vi "Check Mouse In Border Focus.vi"(8 "error in (no error)":errorcluster, 10 "MousePoint":cluster{"x":i16, "y":i16}, 11 "Canvas in":refnum<class "Canvas.lvclass">) -> (0 "error out":errorcluster, 2 "In Border Focus":bool, 3 "Canvas out":refnum<class "Canvas.lvclass">)   [LabVIEW 2015, in "Canvas.lvclass"]
uses:
  Canvas.lvclass
  Canvas.lvclass/Canvas.ctl
  Scalable Border/Scalable Border.lvclass
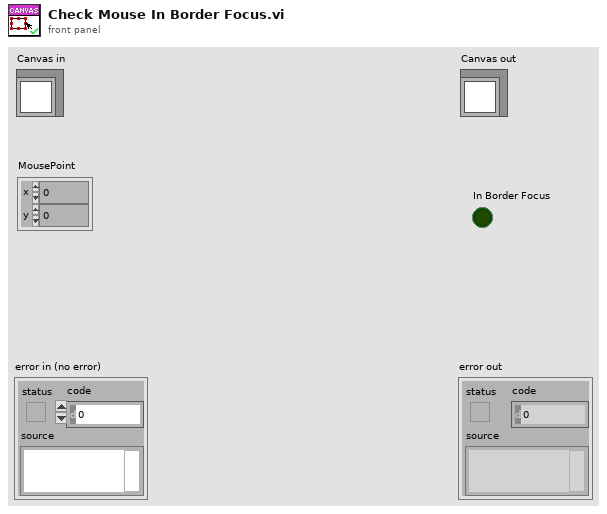
[diagram p1: front panel]
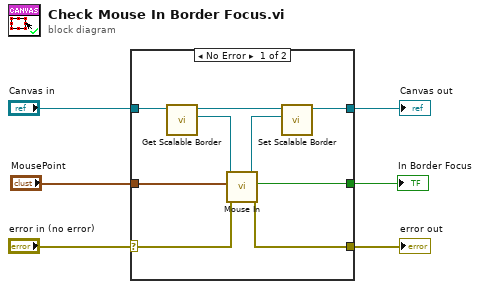
[diagram p0: block diagram]
diagram:
  n1 = case shown="No Error" "error in (no error)" {
    selector: "error in (no error)" -> [w8 w17]
    tunnel: [w7 w17] -> w5
    tunnel: [w10 w16] -> w3
    tunnel: "Canvas in" -> [w15 w16]
    tunnel: "MousePoint" -> [w12 _]
    tunnel: [w11 _] -> w1
    frame No Error {
      n2 = call "Get Scalable Border.vi"("Canvas in"=w15) -> ("Scalable Border"=w13:refnum<class "Scalable Border.lvclass">, "Canvas out"=w14:refnum<class "Canvas.lvclass">)  [unwired: 8 in, 1 out]
      n3 = call-dynamic "Mouse In.vi"("error in (no error)"=w8, "MousePoint"=w12, "Scalable Border in"=w13) -> ("error out"=w7:errorcluster, "In?"=w11:bool, "Scalable Border out"=w9:refnum<class "Scalable Border.lvclass">)  [unwired: 6 in]
      n4 = call "Set Scalable Border.vi"("Scalable Border"=w9, "Canvas in"=w14) -> ("Canvas out"=w10:refnum<class "Canvas.lvclass">)  [unwired: 8 in, 1 out]
    }
    frame Error {
    }
  }
  "error out" <- w5
  "Canvas out" <- w3
  "In Border Focus" <- w1
